vi "SLSC Convert Properties to Tree Control.vi"(4 "string enums":T2(array[cluster]), 6 "Item Indent":i32, 9 "Init Values":variant[](array[variant]), 10 "properties":T3[](array[typedef]), 11 "Child Tag":string) -> (3 "Tree Items":T4(array[cluster]))   [LabVIEW 2017, in "SLSC Tree Control.lvlib"]
doc: "Convert the properties and commands datatypes to a Tree Control items."
uses:
  SLSC Tree Control.lvlib
  Ctrl/Property.ctl
  Ctrl/EnumValue.ctl
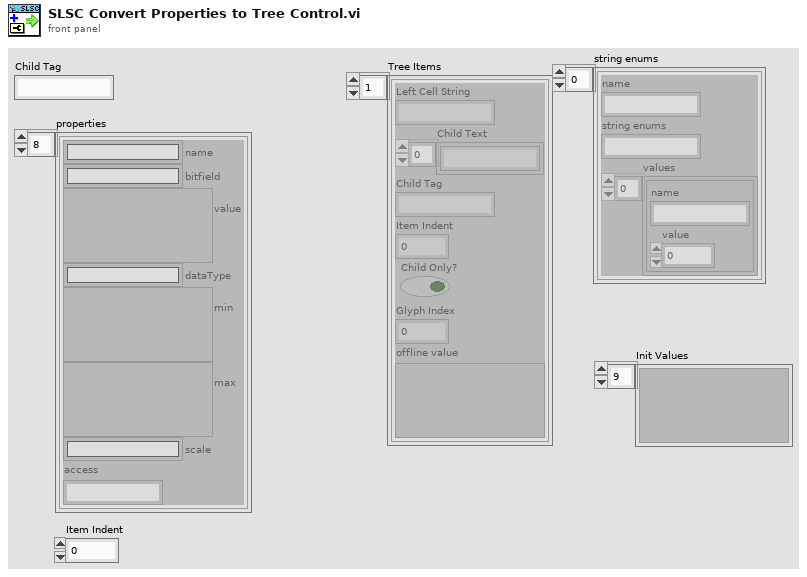
[diagram p1: front panel]
types:
  T1 = typedef "EnumValue.ctl" = cluster{"name":string, "value":i32}
  T2 = cluster{"name":string, "string enums":string, "values":T1[]}[]
  T3 = typedef "Property.ctl" = cluster{"name":string, "bitfield":string, "value":variant, "dataType":string, "min":variant, "max":variant, "scale":string, "access":string}
  T4 = cluster{"Left Cell String":string, "Child Text":string[], "Child Tag":string, "Item Indent":i32, "Child Only?":bool, "Glyph Index":i32, "offline value":variant}[]
  T5 = cluster{"Left Cell String":string, "Child Text":string[], "Child Tag":string, "Item Indent":i32, "Child Only?":bool, "Glyph Index":i32, "offline value":variant}
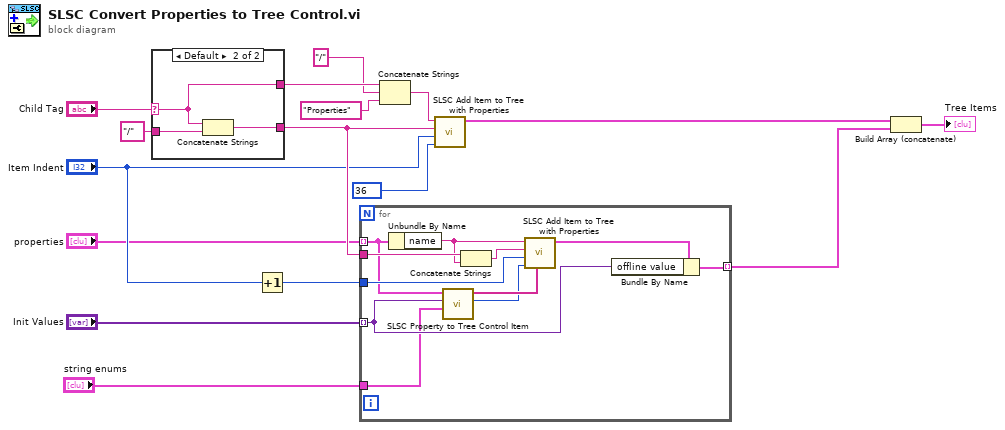
[diagram p0: block diagram]
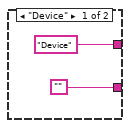
[diagram p2: hidden frame]
diagram:
  n1 = case shown="Default" "Child Tag" {
    selector: "Child Tag" -> [_ w19]
    tunnel: "/" ("string") -> [_ w21]
    tunnel: ["" w20] -> w13
    tunnel: ["Device" ("Left Cell String") w19] -> w4
    frame "Device" {
    }
    frame Default {
      n2 = Concatenate Strings(w19, w21) -> (w20:string)
    }
  }
  n3 = Increment(x="Item Indent") -> (x+1=w12:i32)
  n4 = for {
    tunnel: w13 -> [w32]
    tunnel: [w24] -> w16 mode=indexing
    tunnel: "properties" -> [w29] mode=indexing
    tunnel: w12 -> [w31]
    tunnel: "string enums" -> [w23]
    tunnel: "Init Values" -> [w25] mode=indexing
    n5 = Unbundle By Name(w29) -> ("name"=w22:string)
    n6 = call "SLSC Property to Tree Control Item.vi"("string enums"=w23, "Init value"=w25, "property"=w29) -> ("Glyph"=w27:i32, "Child Text"=w28:string[])  [unwired: 7 in]
    n7 = Concatenate Strings(w32, w22) -> (w30:string)
    n8 = call "SLSC Add Item to Tree with Properties.vi"("Child Text"=w28, "Glyph Index"=w27, "Item indent"=w31, "Child Tag"=w30, "Left Cell String"=w22) -> ("Item"=w26:T5)  [unwired: 6 in]
    n9 = Bundle By Name(cluster=w26, "offline value"=w25) -> (w24:T5)
  }
  n10 = Concatenate Strings(w4, "/" ("string"), "Properties" ("string")) -> (w2:string)
  n11 = call "SLSC Add Item to Tree with Properties.vi"("Glyph Index"=36, "Item indent"="Item Indent", "Child Tag"=w13, "Left Cell String"=w2) -> ("Item"=w15:T5)  [unwired: 7 in]
  n12 = Build Array (concatenate)(w15, w16) -> (→"Tree Items":T4)
